vi "Append Array Element.vi"(8 "error in (no error)":errorcluster, 9 "JSON Value in":refnum<class "JSON Value.lvclass">, 11 "JSON Value in":refnum<class "JSON Value.lvclass">) -> (0 "error out":errorcluster, 2 "JSON Value out":refnum<class "JSON Value.lvclass">)   [LabVIEW 2016, in "JSON Value.lvclass"]
doc: "Appends an array element to an existing JSON Array"
uses:
  JSON Value.lvclass
  JSON Value.lvclass/JSON Value.ctl
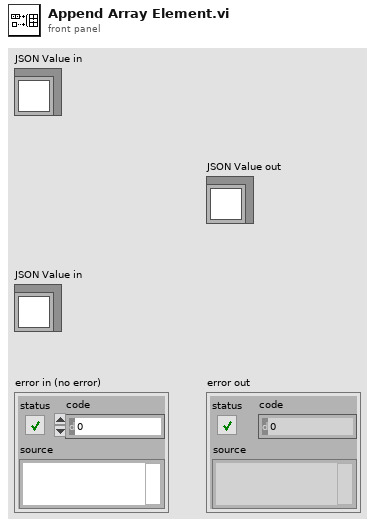
[diagram p1: front panel]
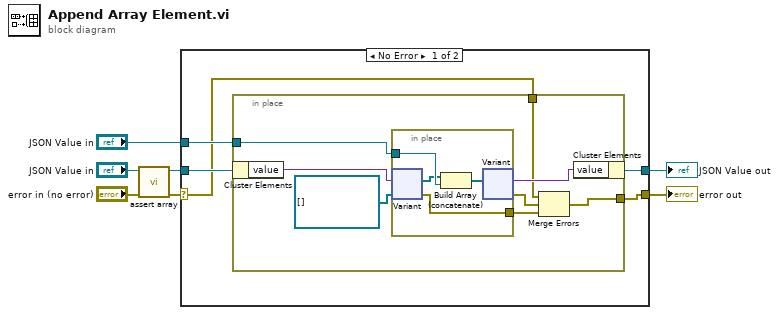
[diagram p0: block diagram]
diagram:
  n1 = call "assert array.vi"("error in (no error)"="error in (no error)", "JSON Value in"="JSON Value in") -> ("error out"=w4:errorcluster, "JSON Value out"=w2:refnum<class "JSON Value.lvclass">)  [unwired: 8 in]
  n2 = case shown="No Error" w4 {
    selector: w4 -> [w8 w25]
    tunnel: w2 -> [w12 w26]
    tunnel: [w11 w26] -> w7
    tunnel: "JSON Value in" -> [w10 _]
    tunnel: [w9 w25] -> w1
    frame No Error {
      n3 = in-place {
        in-place-border: w10 -> [w20]
        in-place-border: [w14] -> w9
        in-place-border: w8 -> [w13]
        n4 = in-place-cluster #1(w12) -> ("value"=w19:variant)
        n5 = in-place {
          in-place-border: w20 -> [w24]
          in-place-border: [w21] -> w15
          n6 = in-place-variant #2(w19, refnum<class "JSON Value.lvclass">[] [] ("JSON Array in")) -> (w23:refnum<class "JSON Value.lvclass">[], w21:errorcluster)
          n7 = Build Array (concatenate)(w23, w24) -> (w22:refnum<class "JSON Value.lvclass">[])
          n8 = in-place-variant #2(w22) -> (w17:variant, w16:errorcluster)
        }
        n9 = Merge Errors(w13, w16, w15) -> (w14:errorcluster)
        n10 = in-place-cluster #1("value"=w17) -> (w11:refnum<class "JSON Value.lvclass">)
      }
    }
    frame Error {
    }
  }
  "JSON Value out" <- w7
  "error out" <- w1
